vi "data-center-simulator.vi"() -> ()   [LabVIEW 2024]
uses:
  <vilib>/Utility/error.llb/DialogType.ctl
  <vilib>/DAQmx/write.llb/DAQmx Write (Analog 1D Wfm NChan NSamp).vi
  <vilib>/DAQmx/create/channels.llb/DAQmx Create Channel (AO-Voltage-Basic).vi
  <vilib>/DAQmx/configure/timing.llb/DAQmx Timing (Sample Clock).vi
  <vilib>/DAQmx/miscellaneous.llb/DAQmx Fill In Error Info.vi
  <resource>/objmgr/daqmx.rc
panel:
  in  "Tab Control":T1(tab)=enum."Power Signals"
  in  "Maximum Value":dbl=10.0 format="%0.2f"
  in  "Minimum Value":dbl=-10.0 format="%0.2f"
  in  "Physical Channels":tag="voltage-output/ao0:2, current-output/ao0:2"
  in  "Sample Clock Rate":dbl=20000.0 format="%0.2f"
  out "Actual Sample Clock Rate":dbl=20000.0 format="%.2f"
  in  "Harmonics":T2(array[cluster])=[[{"level (%)"=0.0, "phase (°)"=0.0, "harm."=1.0}], [{"level (%)"=0.0, "phase (°)"=0.0, "harm."=1.0}], [{"level (%)"=0.0, "phase (°)"=0.0, "harm."=1.0}], [{"level (%)"=0.0, "phase (°)"=0.0, "harm."=1.0}], [{"level (%)"=0.0, "phase (°)"=0.0, "harm."=1.0}], [{"level (%)"=0.0, "phase (°)"=0.0, "harm."=1.0}]]
  in  "Fundamental":cluster{"level (%)":dbl, "phase (°)":dbl}[](array[cluster])=[{"level (%)"=100.0, "phase (°)"=0.0}, {"level (%)"=100.0, "phase (°)"=120.0}, {"level (%)"=100.0, "phase (°)"=240.0}, {"level (%)"=5.0, "phase (°)"=5.0}, {"level (%)"=5.0, "phase (°)"=125.0}, {"level (%)"=5.0, "phase (°)"=245.0}]
  in  "Frequency and Amplitude":T3={"frequency (Hz)"=60.0, "voltage (V) RMS"=7.0, "current (A) RMS"=1.0} {"current (A) RMS" scale=0.0..1.0; "voltage (V) RMS" scale=0.0..7.0; "frequency (Hz)" scale=40.0..60.0}
  out "System Waveform Graph":waveform(dbl)[](graph) caption="Output Waveform"
  in  "inject-spikes":bool
  in  "inject-harmonic":bool
  in  "Injected Harmonic Variables":T4(array[cluster])=[{"level (%)"=0.1, "phase (°)"=330.0, "harm."=3.0}]
  in  "Injected Harmonic Placement":i32=3
  in  "stop":bool
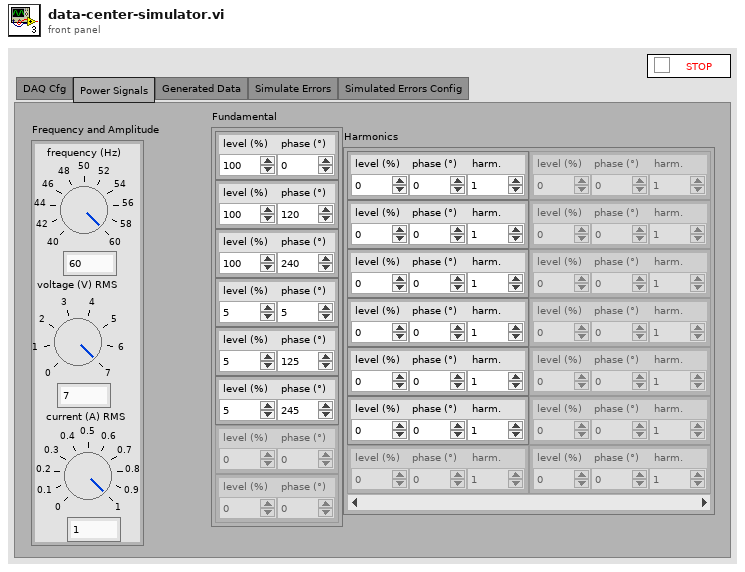
[diagram p1: front panel]
types:
  T1 = enum32{"DAQ Cfg", "Power Signals", "Generated Data", "Simulate Errors", "Simulated Errors Config"}
  T2 = cluster{"level (%)":dbl, "phase (°)":dbl, "harm.":dbl}[][]
  T3 = cluster{"frequency (Hz)":sgl, "voltage (V) RMS":dbl, "current (A) RMS":dbl}
  T4 = cluster{"level (%)":dbl, "phase (°)":dbl, "harm.":dbl}[]
  T5 = typedef "DialogType.ctl" = u16
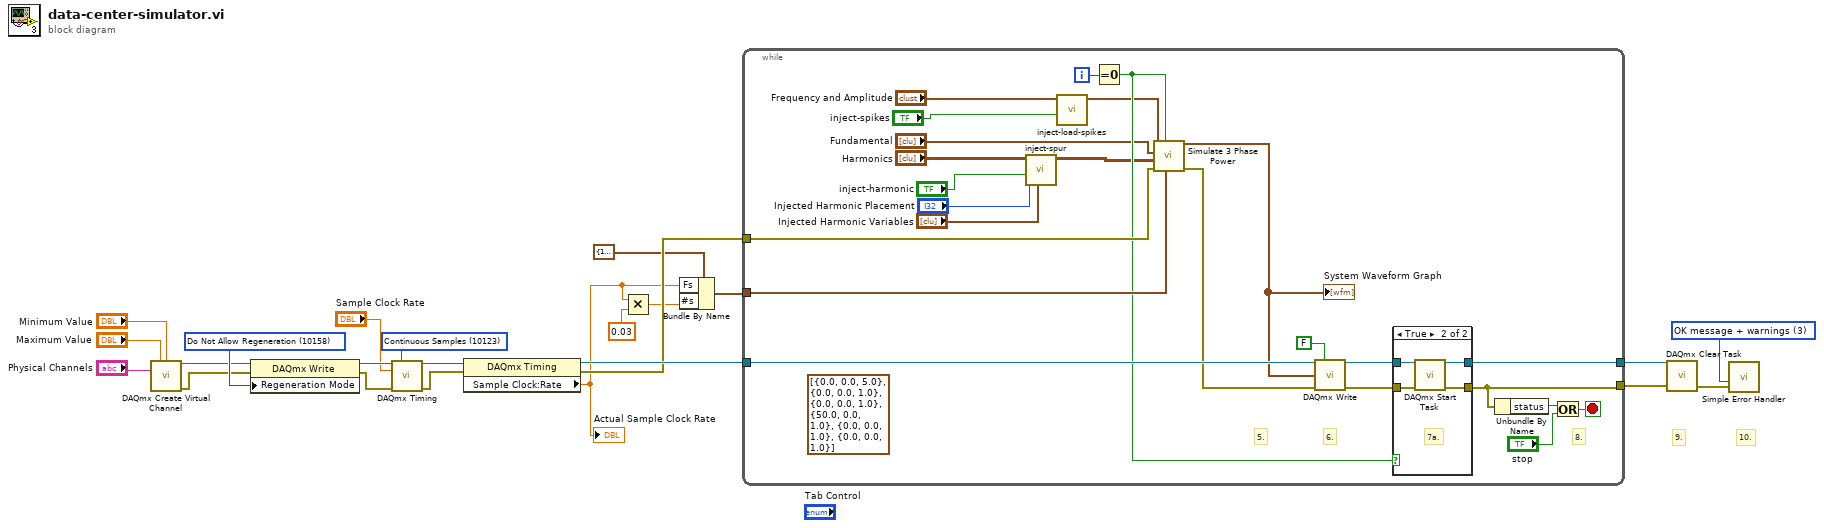
[diagram p0: block diagram]
diagram:
  w13 = 10158 items=["Allow Regeneration"=10097, "Do Not Allow Regeneration"=10158] ("RegenMode")
  w18 = T5 3 items=["no dialog", "OK message", "continue or stop message", "OK message + warnings", "continue/stop + warnings"] ("type of dialog (OK msg:1)")
  w22 = 10123 items=["Finite Samples"=10178, "Continuous Samples"=10123] ("sample mode")
  # "10."
  # "9."
  n1 = call-poly <vilib>:"DAQmx Create Virtual Channel.vi"("maximum value"="Maximum Value", "minimum value"="Minimum Value", "physical channels"="Physical Channels") -> ("task out"=w12:refnum<k21>, "error out"=w11:errorcluster)  [unwired: 11 in]
  n2 = property class="DAQmx Write"(reference=w12, error in=w11, "Regeneration Mode"=w13) -> (reference out=w9:refnum<k21>, error out=w8:errorcluster)
  n3 = call-poly <vilib>:"DAQmx Timing.vi"("task/channels in"=w9, "sample mode"=w22, "rate"="Sample Clock Rate", "error in"=w8) -> ("task out"=w15:refnum<k21>, "error out"=w14:errorcluster)  [unwired: 10 in]
  n4 = property class="DAQmx Timing"(reference=w15, error in=w14) -> (reference out=w10:refnum<k21>, error out=w6:errorcluster, "Sample Clock:Rate"=w3:dbl)
  "Actual Sample Clock Rate" <- w3
  n5 = Multiply(x=w3, y=0.03) -> (x*y=w2:dbl)
  n6 = Bundle By Name(cluster=cluster{"Fs":dbl, "#s":dbl} {"Fs"=1000.0, "#s"=1000.0} ("sampling info"), "Fs"=w3, "#s"=w2) -> (w4:cluster{"Fs":dbl, "#s":dbl})
  n7 = while {
    tunnel: w10 -> [w44]
    tunnel: [w40] -> w17
    tunnel: [w41] -> w16
    tunnel: w6 -> [w38]
    tunnel: w4 -> [w36]
    i -> [w34]
    stop <- w47 stop-if-true
    (unwired) T2 [[{"level (%)"=0.0, "phase (°)"=0.0, "harm."=5.0}], [{"level (%)"=0.0, "phase (°)"=0.0, "harm."=1.0}], [{"level (%)"=0.0, "phase (°)"=0.0, "harm."=1.0}], [{"level (%)"=50.0, "phase (°)"=0.0, "harm."=1.0}], [{"level (%)"=0.0, "phase (°)"=0.0, "harm."=1.0}], [{"level (%)"=0.0, "phase (°)"=0.0, "harm."=1.0}]] ("Harmonics")
    # "8."
    # "6."
    # "5."
    n8 = call "inject-spur.vi"("Harmonics in"="Injected Harmonic Variables", "inject-harmonic"="inject-harmonic", "index (row)"="Injected Harmonic Placement", "Harmonics 3"="Harmonics") -> ("Harmonics out"=w27:T2)  [unwired: 7 in]
    n9 = call "inject-load-spikes.vi"("inject-spikes"="inject-spikes", "Frequency and Amplitude In"="Frequency and Amplitude") -> ("Frequency and Amplitude Out"=w25:T3)  [unwired: 9 in]
    n10 = Equal To 0?(x=w34) -> (x = 0?=w33:bool)
    n11 = call "Simulate 3 Phase Power.vi"("sampling info"=w36, "Reset"=w33, "error in"=w38, "Harmonics Array"=w27, "Fundamental Array"="Fundamental", "Frequency and Amplitude"=w25) -> ("error out"=w39:errorcluster, "Wfm data"=w37:waveform(dbl)[])  [unwired: 4 in]
    "System Waveform Graph" <- w37
    n12 = call-poly <vilib>:"DAQmx Write.vi"("task/channels in"=w44, "auto start"=FALSE, "data"=w37, "error in"=w39) -> ("task out"=w43:refnum<k21>, "error out"=w42:errorcluster)  [unwired: 9 in, 1 out]
    n13 = case shown="True" w33 {
      tunnel: w43 -> [w49 w53]
      tunnel: w42 -> [w48 w52]
      tunnel: [w48 w51] -> w41
      tunnel: [w49 w50] -> w40
      frame False {
        # "7b."
      }
      frame True {
        # "7a."
        n14 = call <vilib>:"DAQmx Start Task.vi"("task/channels in"=w53, "error in"=w52) -> ("task out"=w50:refnum<k21>, "error out"=w51:errorcluster)  [unwired: 12 in]
      }
    }
    n15 = Unbundle By Name(w41) -> ("status"=w46:bool)
    n16 = Or(x=w46, y="stop") -> (x .or. y?=w47:bool)
  }
  n17 = call <vilib>:"DAQmx Clear Task.vi"("task in"=w17, "error in"=w16) -> ("error out"=w23:errorcluster)  [unwired: 13 in]
  n18 = call <vilib>:"Simple Error Handler.vi"("type of dialog (OK msg:1)"=w18, "error in (no error)"=w23) -> ()  [unwired: 3 in, 5 out]
